vi "MatchStatistic.vi"() -> (0 "Map matching":map{string, i32}(c390), 3 "Matches":i32[](array[numeric]), 8 "Matching array":u64[](array[numeric]))   [LabVIEW 2023]
uses:
  <vilib>/Utility/file.llb/Read Delimited Spreadsheet (string).vi
panel:
  out "Number Matches":dbl[](array[numeric])
  out "Number":dbl[](array[numeric])
  out "Waveform Chart":i32[](graph)
  out "Matches array":i64[][](array[numeric])
  out "tmpResults":dbl[][](array[numeric])
  out "tmpOFRes":i32[](array[numeric])
  # "Колко пъти съвпаденията\nот 1 до 6 се срещат в тиражите до сега"
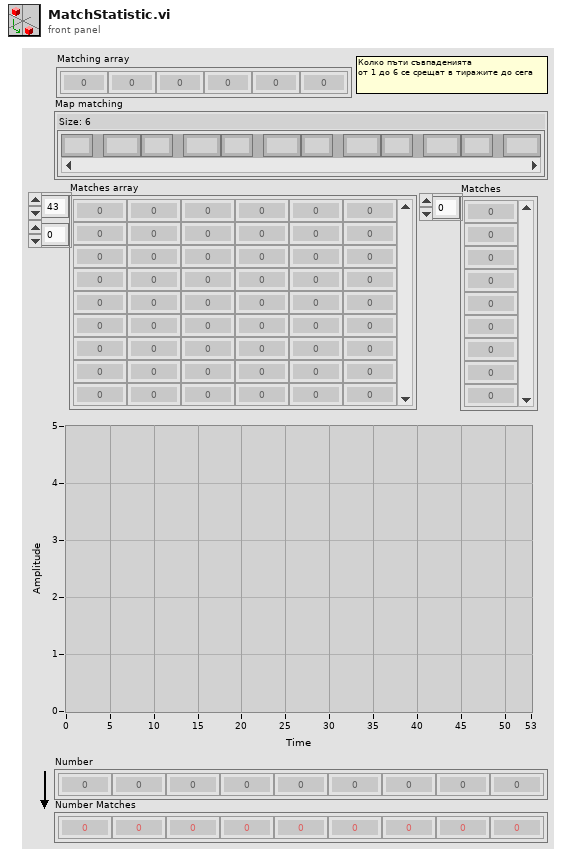
[diagram p1: front panel]
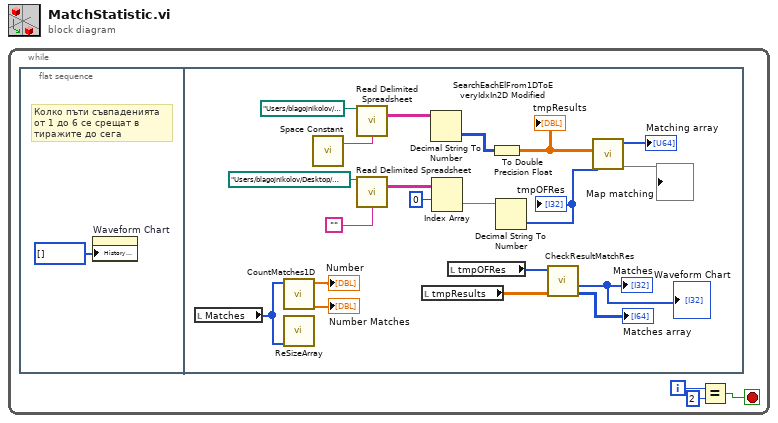
[diagram p0: block diagram]
diagram:
  n1 = while {
    i -> [w3]
    stop <- w1 stop-if-true
    n2 = flat-sequence {
      frame #0 {
        # "Колко пъти съвпаденията\nот 1 до 6 се срещат в \nтиражите до сега"
        n3 = property on="Waveform Chart" class="WFChart (strict)"("History Data"=i32[] []) -> ()  [unwired: 2 in, 2 out]
      }
      frame #1 {
        n4 = local read "Matches"() -> (w7:i32[])
        n5 = call "CountMatches1D.vi"("Array"=w7) -> ("Result"=→"Number Matches":dbl[], "History"=→"Number":dbl[])  [unwired: 9 in]
        n6 = call "ReSizeArray.vi"("1D"=w7) -> ()  [unwired: 9 in, 2 out]
        n7 = call <vilib>:"Space Constant.vi"() -> ("String"=w23:string)
        n8 = call-poly <vilib>:"Read Delimited Spreadsheet.vi"("file path (dialog if empty)"=path "/Users/blagojnikolov/Desktop/@tmp/results.txt", "delimiter (\\t)"=w23) -> ("all rows"=w22:string[][])  [unwired: 8 in, 5 out]
        n9 = call-poly <vilib>:"Read Delimited Spreadsheet.vi"("file path (dialog if empty)"=path "/Users/blagojnikolov/Desktop/@tmp/officialResults.txt", "delimiter (\\t)"="") -> ("all rows"=w18:string[][])  [unwired: 8 in, 5 out]
        n10 = local read "tmpResults"() -> (w5:dbl[][])
        n11 = Decimal String To Number(string=w22) -> (number=w15:i32[][])  [unwired: 2 in, 1 out]
        n12 = Index Array(array=w18, index (row)=0) -> (element=w16:string[])  [unwired: 1 in]
        n13 = local read "tmpOFRes"() -> (w12:i32[])
        n14 = To Double Precision Float(number=w15) -> (double precision float=w6:dbl[][])
        "tmpResults" <- w6
        n15 = Decimal String To Number(string=w16) -> (number=w14:i32[])  [unwired: 2 in, 1 out]
        "tmpOFRes" <- w14
        n16 = call "CheckResultMatchRes.vi"("Your Suppose"=w5, "Last Draw"=w12) -> ("Matches array"=→"Matches array":i64[][], "Matches"=→"Matches" →"Waveform Chart":i32[])  [unwired: 6 in, 2 out]
        n17 = call "SearchEachElFrom1DToEveryIdxIn2D Modified.vi"("This Array"=w14, "2D Target Array"=w6) -> ("Map matching"=→"Map matching":map{string, i32}, "Matching array"=→"Matching array":u64[])  [unwired: 8 in]
      }
    }
    n18 = Equal?(x=w3, y=2) -> (x = y?=w1:bool)
  }
